vi "TDT-Coerce Sampling Rate.vi"(1 "Fs (Hz)":dbl) -> (0 "Coerced":dbl format="%#_10g")   [LabVIEW 2020]
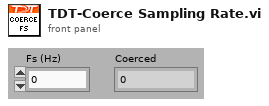
[diagram p1: front panel]
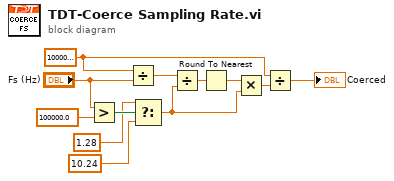
[diagram p0: block diagram]
diagram:
  w11 = 1000000.0 ("x")
  n1 = Greater?(x="Fs (Hz)", y=100000.0) -> (0:w4:bool)
  n2 = Divide(x=w11, y="Fs (Hz)") -> (x/y=w7:dbl)
  n3 = Select(t=1.28 ("y"), s=w4, f=10.24 ("y")) -> (s? t:f=w3:dbl)
  n4 = Divide(x=w7, y=w3) -> (x/y=w8:dbl)
  n5 = Round To Nearest(number=w8) -> (nearest integer value=w9:dbl)
  n6 = Multiply(x=w9, y=w3) -> (x*y=w10:dbl)
  n7 = Divide(x=w11, y=w10) -> (x/y=→"Coerced":dbl)
